vi "DeQueue Action.vi"(0 "action queue in":refnum<queue>, 7 "termination list ([Exit])":string[](array[string])=["Exit"], 9 "timeout in ms (0)":i32, 11 "error in":errorcluster) -> (3 "exit?":bool, 4 "action queue out":refnum<queue>, 6 "action":string, 8 "action value":string, 10 "timed out?":bool, 15 "error out":errorcluster)   [LabVIEW 2016, in "TLB` Template.lvlib" / "Actions.lvlib"]
doc: "Removes an element from the front of a queue and returns the element.\n\n<B>Input Parameters</B>\n\n<B>action queue in</B> is a reference to a queue. Use the Create Action Queue function to obtain a queue reference. \n\n<B>termination list</B> is a list of actions that end the action queue.\n\n<B>timeout (ms)</B> trigger queue timeout.\n\n<B>error in</B> describes error conditions that occur before this node runs. This input provides standard error in functionality.\n\n<B>Output Parameters</B>\n\n<B>action queue out</B> returns the reference to the queue unchanged. \n\n<B>action</B> available system action.\n\n<B>action value/B> data action as part of the system action.\n\n<B>error out</B> contains error information. This output provides standard error out functionality."
uses:
  Actions.lvlib
  System Action Element.ctl
  <vilib>/regexp/Match Regular Expression.xnode
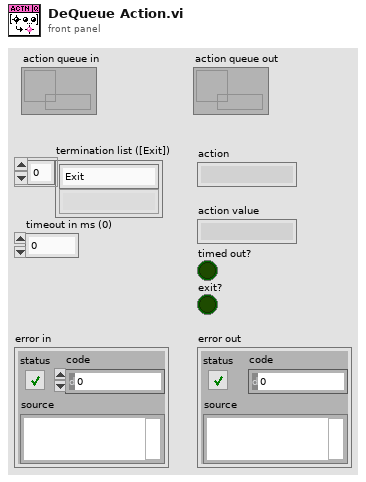
[diagram p1: front panel]
types:
  T1 = typedef "TLB` Template.lvlib/Actions.lvlib/System Action Element.ctl" = cluster{"action":string, "data":string}
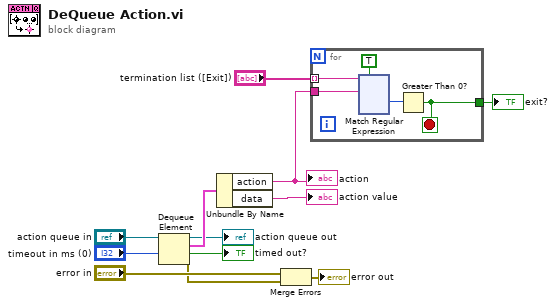
[diagram p0: block diagram]
diagram:
  n1 = Dequeue Element(queue="action queue in", timeout in ms (-1)="timeout in ms (0)") -> (queue out=→"action queue out":refnum<queue>, element=w12:T1, timed out?=→"timed out?":bool, error out=w6:errorcluster)  [unwired: 1 in]
  n2 = Unbundle By Name(w12) -> ("action"=w9:string, "data"=→"action value":string)
  "action" <- w9
  n3 = Merge Errors("error in", w6) -> (→"error out":errorcluster)
  n4 = for {
    tunnel: "termination list ([Exit])" -> [w17] mode=indexing
    tunnel: w9 -> [w16]
    tunnel: [w13] -> w8
    stop <- w13 stop-if-true
    n5 = xnode "Match Regular Expression"("input string"=w17, "regular expression"=w16, "ignore case? (F)"=TRUE) -> ("offset past match"=w14:i32)  [unwired: 3 in, 4 out]
    n6 = Greater Than 0?(x=w14) -> (x > 0?=w13:bool)
  }
  "exit?" <- w8
